vi "initialize.vi"(8 "ErrorIn":errorcluster) -> (0 "ErrorOut":errorcluster, 3 "Queues":T1)   [LabVIEW 2019]
uses:
  utilities/AQueues.ctl
  UIVIs/AccelerationDataFrames.ctl
  AmasterVIs/ACommand.ctl
  utilities/AnalyzerSettings.ctl
  AmasterVIs/AThreads.ctl
  utilities/FGVAction.ctl
  UIVIs/UIOutput.ctl
  UIVIs/UIOutputFGVAction.ctl
  AmasterVIs/ACommandQueuesAction.ctl
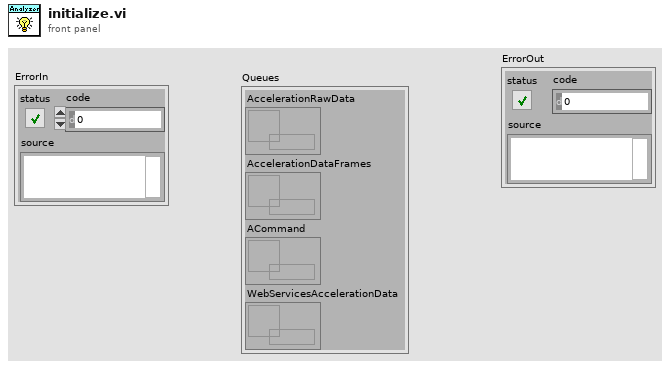
[diagram p1: front panel]
types:
  T1 = typedef "AQueues.ctl" = cluster{"AccelerationRawData":refnum<queue>, "AccelerationDataFrames":refnum<queue>, "ACommand":refnum<queue>, "WebServicesAccelerationData":refnum<queue>}
  T2 = typedef "ACommand.ctl" = enum16{"None", "Start", "Stop", "Restart"}
  T3 = typedef "UIOutputFGVAction.ctl" = enum16{"Read", "Write", "CheckUpdate"}
  T4 = typedef "UIOutput.ctl" = cluster{"Aquiring data":bool, "AnalyzerError":errorcluster, "FIFO overflow":bool, "Analyzing data":bool}
  T5 = typedef "FGVAction.ctl" = enum16{"Read", "Write"}
  T6 = typedef "AnalyzerSettings.ctl" = cluster{"fs [Hz]":dbl, "Create NS Timeout Code":i32, "Destroy NS Timeout Code":i32, "All threads":T7[]}
  T7 = typedef "AThreads.ctl" = enum16{"UI", "analyzeAccelerationData", "aquireAccelerationData", "communicateWebServices"}
  T8 = typedef "ACommandQueuesAction.ctl" = enum16{"Initialize", "Set", "Get", "ReleaseAll"}
  T9 = typedef "AccelerationDataFrames.ctl" = cluster{"AccelerationData":waveform(dbl)[], "Amplitudes":cluster{"f0":dbl, "df":dbl, "real part":dbl[]}[], "Phases":cluster{"f0":dbl, "df":dbl, "imaginary part":dbl[]}[]}
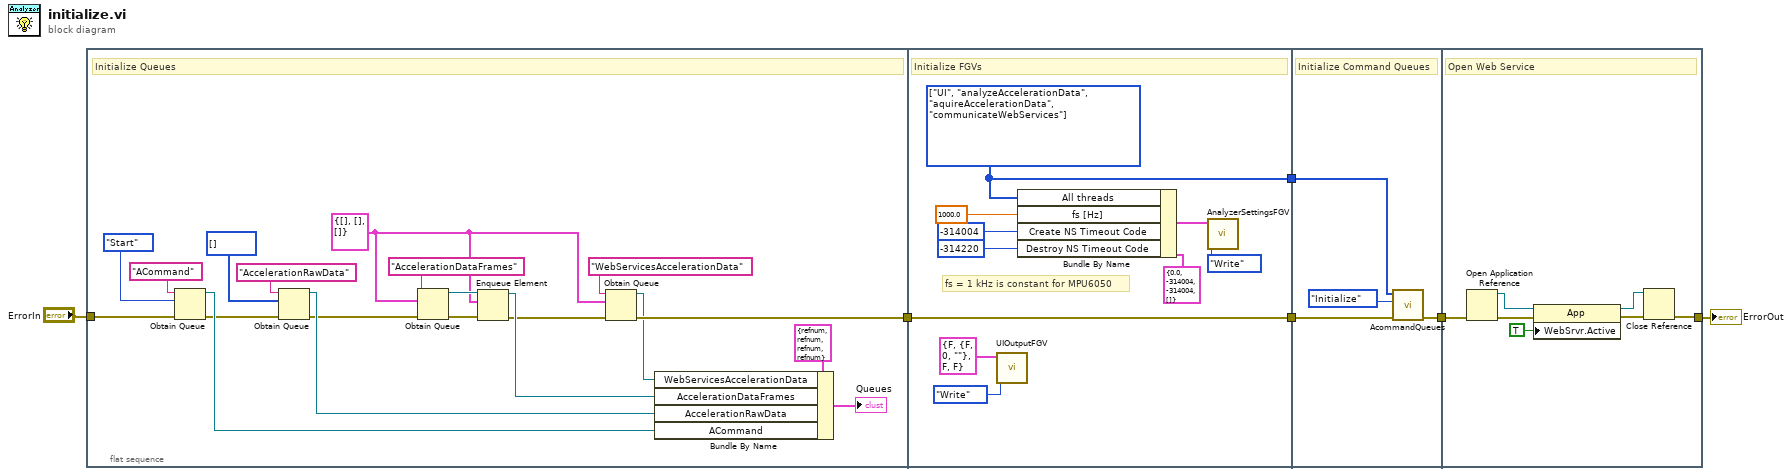
[diagram p0: block diagram]
diagram:
  n1 = flat-sequence {
    tunnel: "ErrorIn" -> [w15]
    tunnel: [w13] -> w5
    tunnel: w5 -> [w32]
    tunnel: [w32] -> w3
    tunnel: [w27] -> w1
    tunnel: w3 -> [w40]
    tunnel: [w39] -> w2
    tunnel: w1 -> [w38]
    tunnel: [w42] -> w4
    tunnel: w2 -> [w47]
    frame #0 {
      w7 = T9 {"AccelerationData"=[], "Amplitudes"=[], "Phases"=[]} ("AccelerationDataFrames")
      # "Initialize Queues"
      n2 = Obtain Queue(name (unnamed)="ACommand", element data type=ACommand."Start" ("AnalyzerCommand"), error in (no error)=w15) -> (queue out=w9:refnum<queue>, error out=w8:errorcluster)  [unwired: 2 in, 1 out]
      n3 = Obtain Queue(name (unnamed)="AccelerationRawData", element data type=u8[] [] ("AccelerationRawData"), error in (no error)=w8) -> (queue out=w26:refnum<queue>, error out=w22:errorcluster)  [unwired: 2 in, 1 out]
      n4 = Obtain Queue(name (unnamed)="AccelerationDataFrames", element data type=w7, error in (no error)=w22) -> (queue out=w21:refnum<queue>, error out=w23:errorcluster)  [unwired: 2 in, 1 out]
      n5 = Enqueue Element(queue=w21, element=w7, error in (no error)=w23) -> (queue out=w25:refnum<queue>, error out=w14:errorcluster)  [unwired: 1 in, 1 out]
      n6 = Obtain Queue(name (unnamed)="WebServicesAccelerationData", element data type=w7, error in (no error)=w14) -> (queue out=w11:refnum<queue>, error out=w13:errorcluster)  [unwired: 2 in, 1 out]
      n7 = Bundle By Name(cluster=T1 {"AccelerationRawData"=refnum, "AccelerationDataFrames"=refnum, "ACommand"=refnum, "WebServicesAccelerationData"=refnum} ("Queues"), "WebServicesAccelerationData"=w11, "AccelerationDataFrames"=w25, "AccelerationRawData"=w26, "ACommand"=w9) -> (→"Queues":T1)
    }
    frame #1 {
      w27 = T7[] [enum."UI", enum."analyzeAccelerationData", enum."aquireAccelerationData", enum."communicateWebServices"] items=["UI", "analyzeAccelerationData", "aquireAccelerationData", "communicateWebServices"] ("All threads")
      # "fs = 1 kHz is constant for MPU6050"
      # "Initialize FGVs"
      n8 = call "UIOutputFGV.vi"("FGVAction (Read)"=UIOutputFGVAction."Write", "UIOutputIn"=T4 {"Aquiring data"=FALSE, "AnalyzerError"={"status"=FALSE, "code"=0, "source"=""}, "FIFO overflow"=FALSE, "Analyzing data"=FALSE}) -> ()  [unwired: 8 in, 2 out]
      n9 = Bundle By Name(cluster=T6 {"fs [Hz]"=0.0, "Create NS Timeout Code"=-314004, "Destroy NS Timeout Code"=-314004, "All threads"=[]} ("GlobalSettings"), "All threads"=w27, "fs [Hz]"=1000.0 ("fs"), "Create NS Timeout Code"=-314004 ("Network Stream Timeout Code"), "Destroy NS Timeout Code"=-314220 ("Read Network Stream Timeout")) -> (w36:T6)
      n10 = call "AnalyzerSettingsFGV.vi"("FGVAction (Read)"=FGVAction."Write" ("FGVAction"), "GlobalSettingsIn"=w36) -> ()  [unwired: 9 in, 1 out]
    }
    frame #2 {
      # "Initialize Command Queues"
      n11 = call "AcommandQueues.vi"("ErrorIn"=w40, "ACommandQueuesAction"=ACommandQueuesAction."Initialize", "AThreads"=w38) -> ("ErrorOut"=w39:errorcluster)  [unwired: 7 in, 1 out]
    }
    frame #3 {
      # "Open Web Service"
      n12 = Open Application Reference(8:w47) -> (0:w46:errorcluster, 3:w45:refnum<vi>)  [unwired: 3 in]
      n13 = property class="App"(reference=w45, error in=w46, "WebSrvr.Active"=TRUE ("Web Server:Server Active")) -> (reference out=w41:refnum<vi>, error out=w43:errorcluster)
      n14 = Close Reference(reference=w41, error in (no error)=w43) -> (error out=w42:errorcluster)
    }
  }
  "ErrorOut" <- w4
